vi "main.vi"(0 "Power":bool, 1 "Bean level":dbl(slide) scale=0.0..100.0, 2 "Milk level":dbl(slide) scale=0.0..100.0, 5 "1 Cup":bool, 7 "1 Carafe":bool, 8 "Chamber":dbl(slide) scale=0.0..60.0, 9 "Water level":dbl(slide) scale=0.0..100.0, 10 "Dispenser":dbl(slide) scale=0.0..60.0, 11 "Error in":errorcluster) -> (4 "Elapsed Time":dbl, 6 "Total Cups":dbl, 12 "Low Water":bool, 13 "Low Bean":bool, 14 "Low Milk":bool, 15 "Error out":errorcluster)   [LabVIEW 2020, in "coffee machine.lvlib"]
doc: "This system is a coffee maker which can be produce variety of coffees based on the user input."
uses:
  coffee machine.lvlib
  Typedefs/Queue operations.ctl
  Typedefs/Data cluster.ctl
  <vilib>/Utility/config.llb/Write Key (String).vi
  <vilib>/Utility/config.llb/NI_LVConfig.lvlib
panel:
  out "Previous time":dbl
  out "Dispensing":bool
  out "Brewing":bool
  out "Grinding":bool
  out "Heating":bool
  out "Purging":bool
  in  "Select drink":dbl(knob) scale=0.0..10.0
  # "Coffee"
  # "Latte"
  # "Hot water"
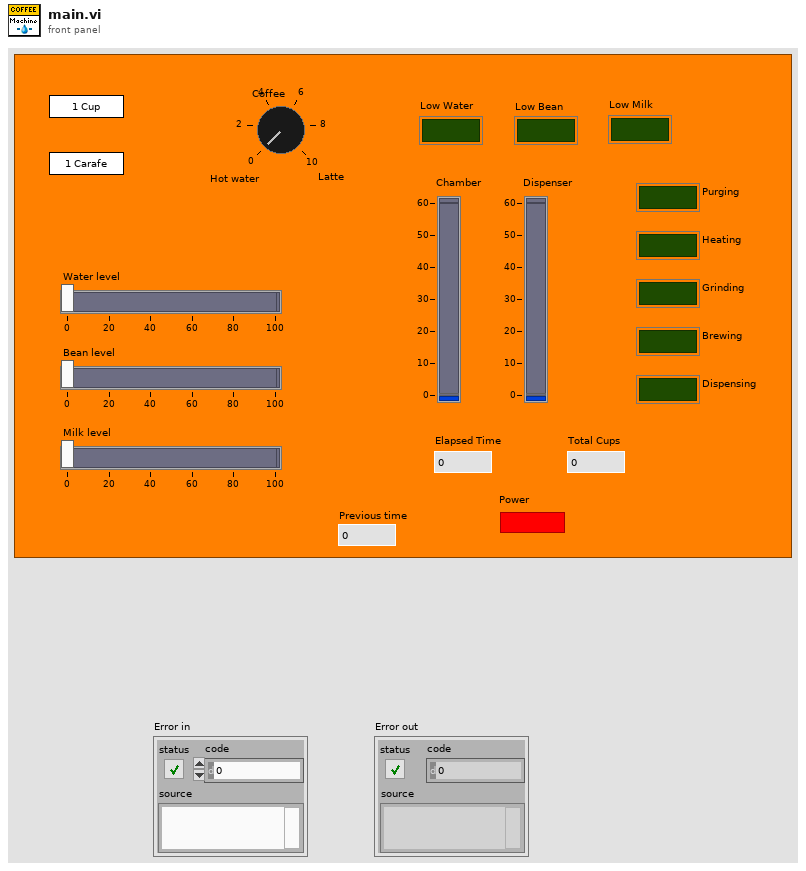
[diagram p1: front panel]
types:
  T1 = typedef "Data cluster.ctl" = cluster{"Timing":cluster{"Start time":dbl, "Elapsed time":dbl, "Previous time":dbl, "Started":bool, "Paused":bool}, "Enable controls":refnum<vi>[], "Disable controls":refnum<vi>[], "Low Water":bool, "Low Bean":bool, "Low Milk":bool, "Purging":bool, "Heating":bool, "Grinding":bool, "Brewing":bool, "Dispensing":bool, "Elapsed time":dbl, "Total Cups":dbl, "Path":path}
  T2 = typedef "coffee machine.lvlib/Queue operations.ctl" = enum16{"Create queue", " Enqueue N", "Enstack N", "Dequeue", "Flush", "Release", ""}
  T3 = cluster{"Start time":dbl, "Elapsed time":dbl, "Previous time":dbl, "Started":bool, "Paused":bool}
  T4 = typedef "NI_LVConfig.lvlib/Config Data RefNum.ctl" = refnum<k1>
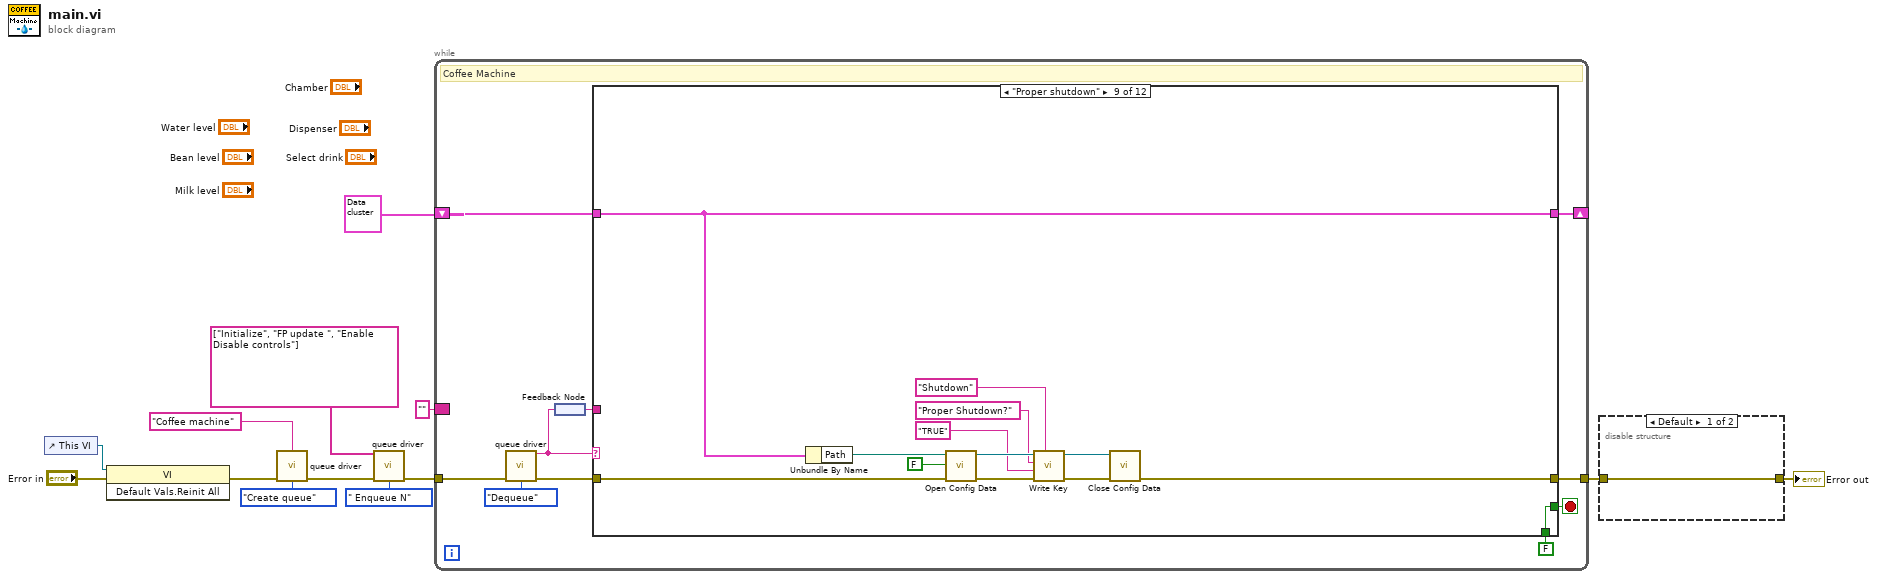
[diagram p0: block diagram]
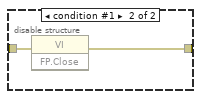
[diagram p2: hidden frame]
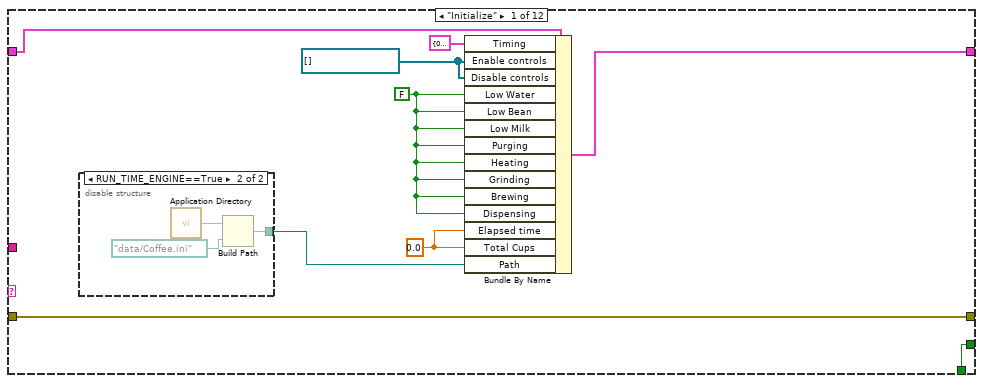
[diagram p3: hidden frame]
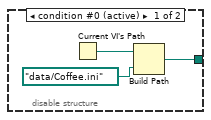
[diagram p4: hidden frame]
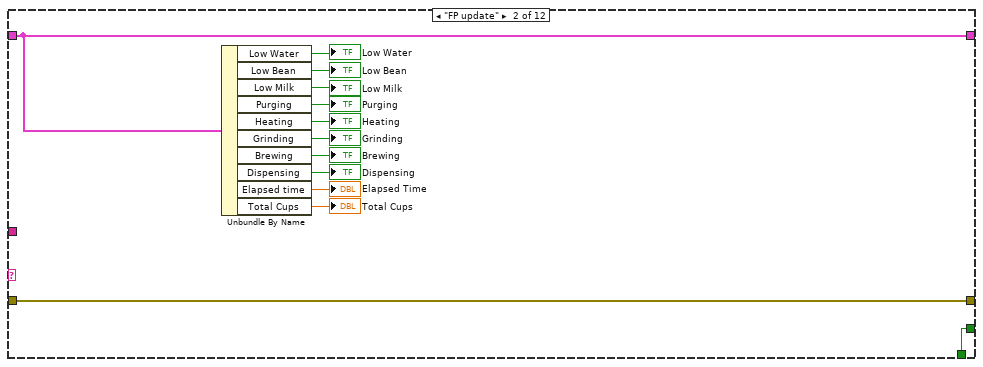
[diagram p5: hidden frame]
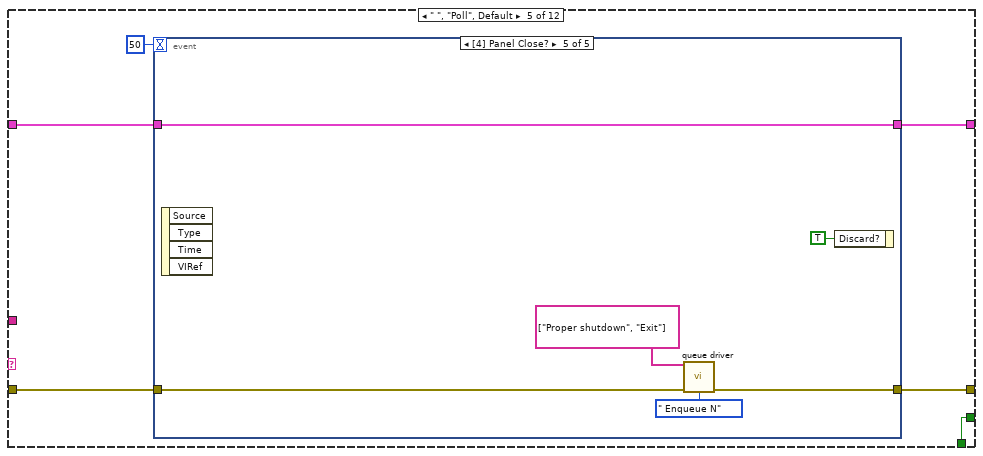
[diagram p8: hidden frame]
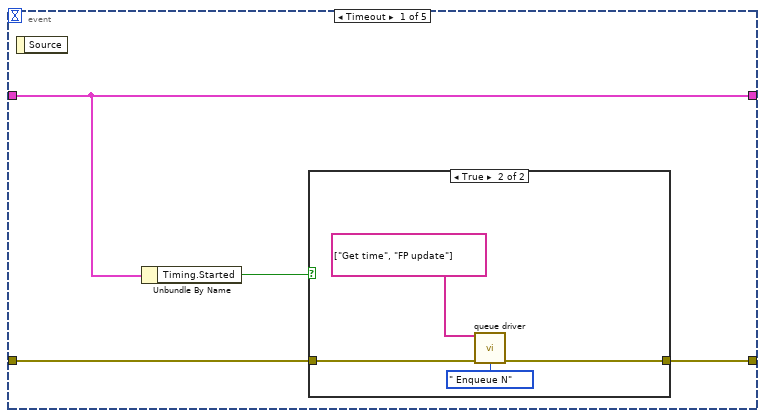
[diagram p9: hidden frame]
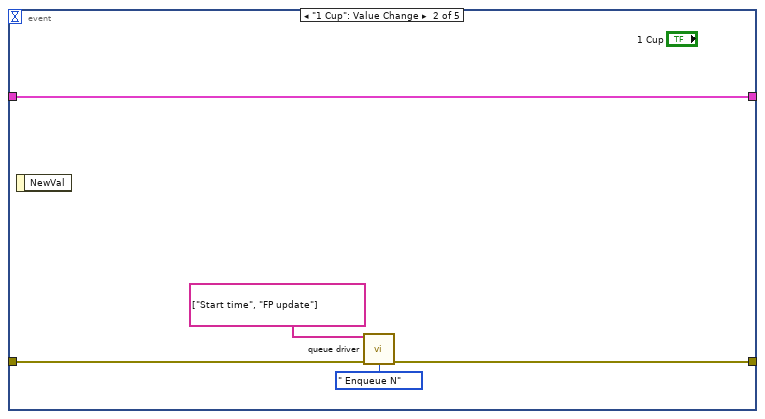
[diagram p11: hidden frame]
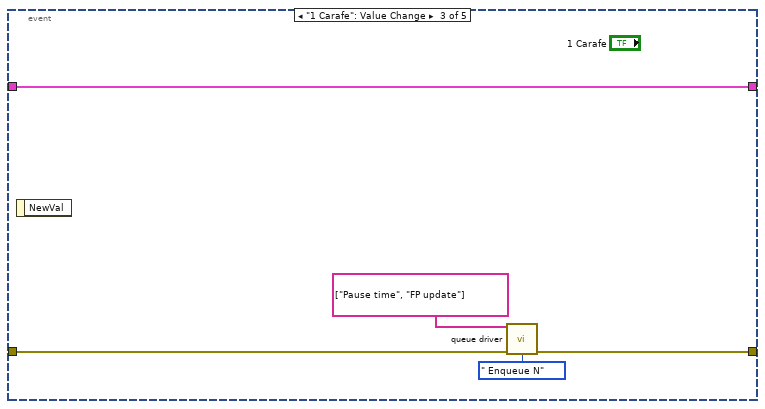
[diagram p12: hidden frame]
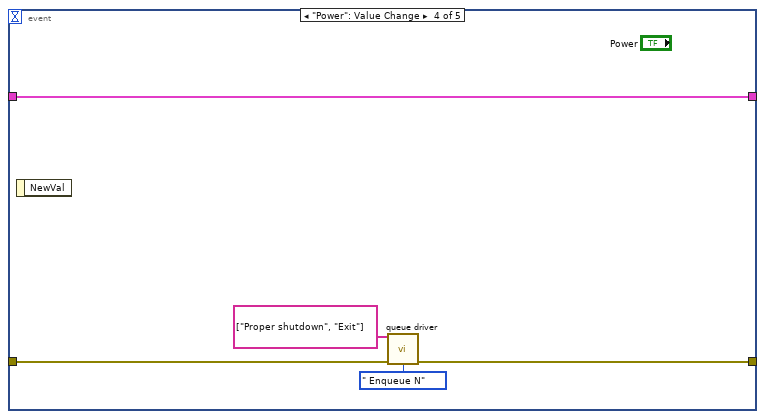
[diagram p13: hidden frame]
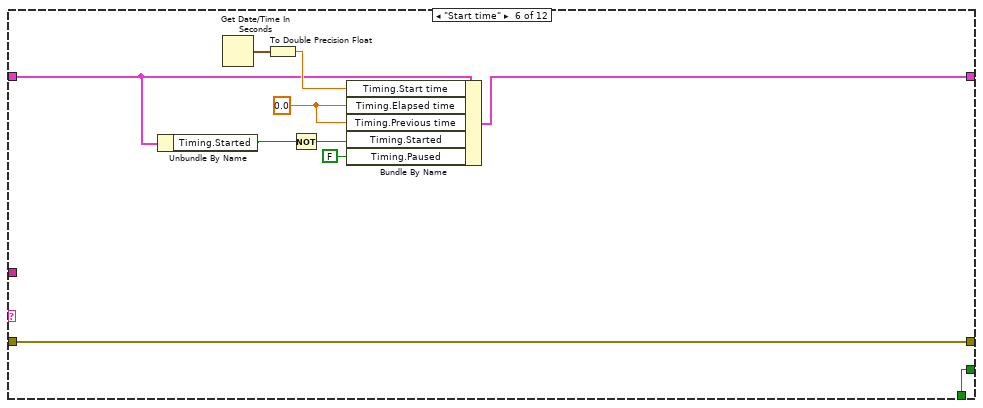
[diagram p14: hidden frame]
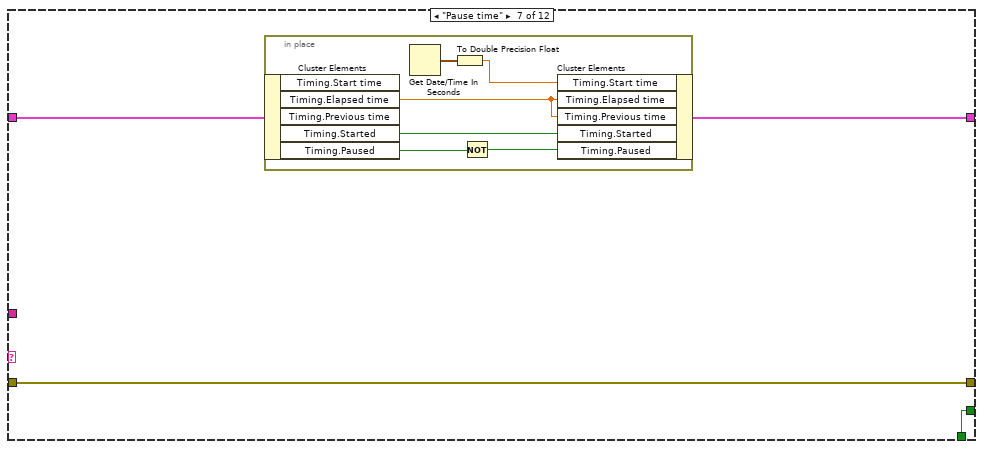
[diagram p15: hidden frame]
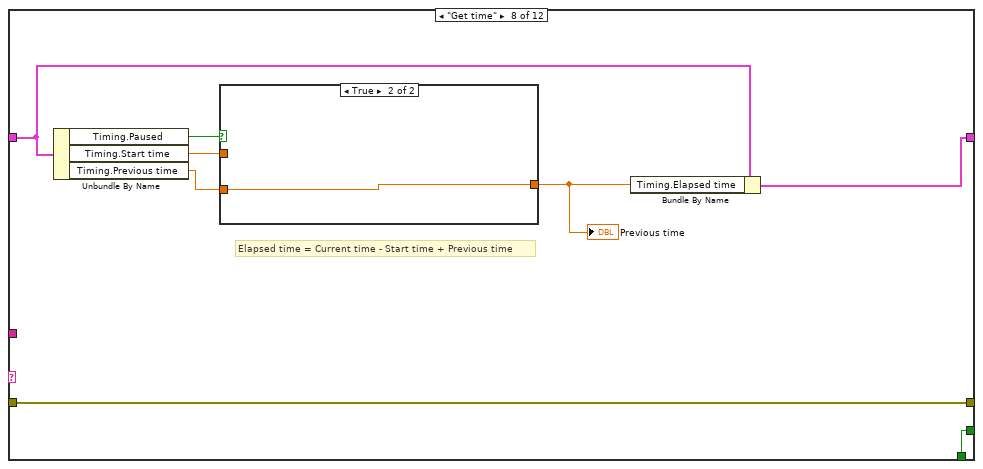
[diagram p16: hidden frame]
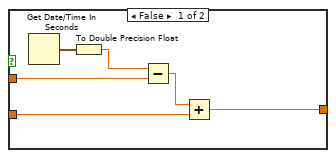
[diagram p17: hidden frame]
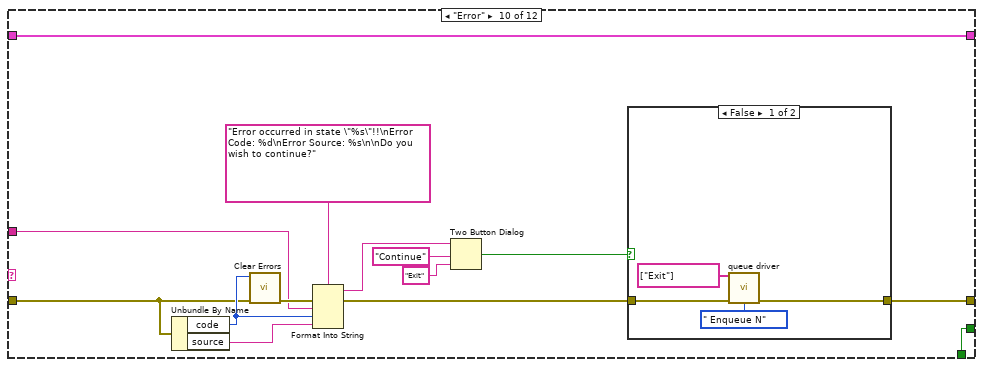
[diagram p18: hidden frame]
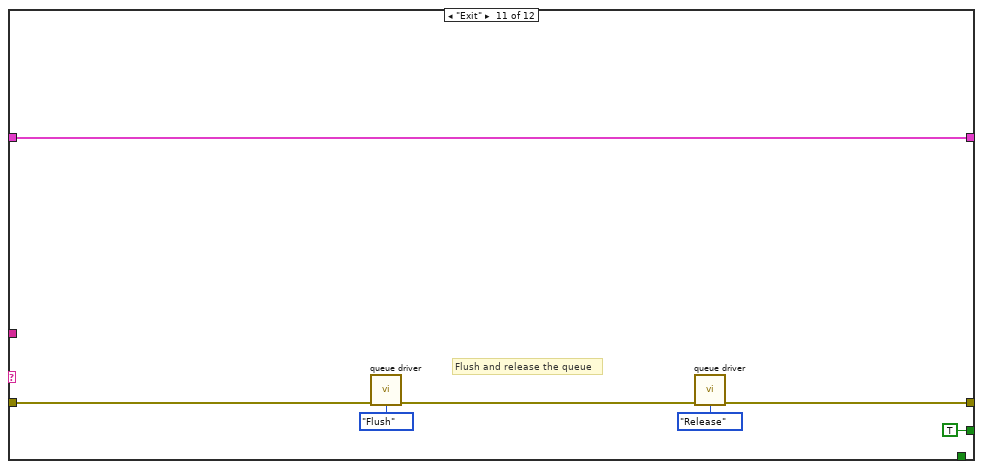
[diagram p20: hidden frame]
diagram:
  n1 = control-ref of="This VI"() -> (w11:refnum<vi>)
  n2 = invoke class="VI" method="Default Vals.Reinit All"(reference=w11, error in="Error in") -> (error out=w10:errorcluster)  [unwired: 1 in, 2 out]
  n3 = call "queue driver.vi"("Name"="Coffee machine", "Error in"=w10, "Queue operations"=Queue_operations."Create queue") -> ("Error out"=w7:errorcluster)  [unwired: 11 in, 1 out]
  n4 = call "queue driver.vi"("Enqueue"=string[] ["Initialize", "FP update ", "Enable Disable controls"], "Error in"=w7, "Queue operations"=Queue_operations." Enqueue N") -> ("Error out"=w5:errorcluster)  [unwired: 11 in, 1 out]
  n5 = while {
    tunnel: w5 -> [w20]
    border: "" ("Dequeued element") -> [_]
    shift-right: [w15] -> _
    shift-left: T1 {"Timing"={"Start time"=0.0, "Elapsed time"=0.0, "Previous time"=0.0, "Started"=FALSE, "Paused"=FALSE}, "Enable controls"=[], "Disable controls"=[], "Low Water"=FALSE, "Low Bean"=FALSE, "Low Milk"=FALSE, "Purging"=FALSE, "Heating"=FALSE, "Grinding"=FALSE, "Brewing"=FALSE, "Dispensing"=FALSE, "Elapsed time"=0.0, "Total Cups"=0.0, "Path"=path ""} -> [w14]
    tunnel: [w16] -> w2
    stop <- w23 stop-if-true
    # "Coffee Machine"
    n6 = call "queue driver.vi"("Error in"=w20, "Queue operations"=Queue_operations."Dequeue") -> ("Dequeued element"=w19:string, "Error out"=w17:errorcluster)  [unwired: 12 in]
    n7 = feedback-in #1(w19) -> ()
    n8 = feedback #1() -> (w18:string)
    n9 = case shown="\"Proper shutdown\"" w19 {
      tunnel: [w32 w51 w54 w57 w63 w103 w107 w121 w141 w155 TRUE w170] -> w23
      tunnel: FALSE -> [w32 w51 w54 w57 w63 w103 w107 w121 w141 w155 _ w170]
      tunnel: w18 -> [_ _ _ _ _ _ _ _ _ w146 _ _]
      tunnel: w17 -> [w31 w50 w53 w56 w62 w102 w106 w120 w140 w147 w165 w169]
      tunnel: [w31 w50 w53 w56 w61 w102 w106 w120 w130 w143 w163 w169] -> w16
      tunnel: [w25 w39 w52 w55 w59 w101 w104 w114 w129 w142 w161 w168] -> w15
      tunnel: w14 -> [w30 w39 w52 w55 w58 w96 w105 w116 w129 w142 w161 w168]
      frame "Initialize" {
        w26 = 0.0 ("Total Cups")
        w27 = FALSE ("Low Water")
        w28 = refnum<vi>[] [] ("Enable controls")
        n10 = disable-structure shown="RUN_TIME_ENGINE==True" {
          disable-tunnel: [w33 w37] -> w24
          frame condition #0 (active) {
            n11 = Current VI's Path() -> (path=w35:path)
            n12 = Build Path(base path=w35, name or relative path=path "data/Coffee.ini") -> (appended path=w33:path)
          }
          frame condition #1 {
            n13 = call <vilib>:"Application Directory.vi"() -> ("Application Directory"=w36:path)
            n14 = Build Path(base path=w36, name or relative path=path "data/Coffee.ini") -> (appended path=w37:path)
          }
        }
        n15 = Bundle By Name(cluster=w30, "Timing"=T3 {"Start time"=0.0, "Elapsed time"=0.0, "Previous time"=0.0, "Started"=FALSE, "Paused"=FALSE}, "Enable controls"=w28, "Disable controls"=w28, "Low Water"=w27, "Low Bean"=w27, "Low Milk"=w27, "Purging"=w27, "Heating"=w27, "Grinding"=w27, "Brewing"=w27, "Dispensing"=w27, "Elapsed time"=w26, "Total Cups"=w26, "Path"=w24) -> (w25:T1)
      }
      frame "FP update" {
        n16 = Unbundle By Name(w39) -> ("Low Water"=→"Low Water":bool, "Low Bean"=→"Low Bean":bool, "Low Milk"=→"Low Milk":bool, "Purging"=→"Purging":bool, "Heating"=→"Heating":bool, "Grinding"=→"Grinding":bool, "Brewing"=→"Brewing":bool, "Dispensing"=→"Dispensing":bool, "Elapsed time"=→"Elapsed Time":dbl, "Total Cups"=→"Total Cups":dbl)
      }
      frame "Enable Disable controls" {
      }
      frame "Read and write file" {
      }
      frame " ", "Poll", Default {
        n17 = event shown="[4] Panel Close?" {
          selector: _ -> [_ _ _ _ _]
          dyn-events: _ -> [_ _ _ _ _]
          timeout: 50 -> [_ _ _ _ _]
          tunnel: w62 -> [w65 w75 w79 w85 w89]
          tunnel: [w64 w74 w78 w84 w88] -> w61
          tunnel: [w67 w77 w82 w87 w93] -> w59
          tunnel: w58 -> [w67 w77 w82 w87 w93]
          event Timeout {
            n18 = event-data() -> ()  [unwired: 1 in, 1 out]
            n19 = Unbundle By Name(w67) -> ("Timing.Started"=w66:bool)
            n20 = case shown="True" w66 {
              tunnel: w65 -> [w68 w71]
              tunnel: [w68 w70] -> w64
              frame False {
              }
              frame True {
                n21 = call "queue driver.vi"("Enqueue"=string[] ["Get time", "FP update"], "Error in"=w71, "Queue operations"=Queue_operations." Enqueue N") -> ("Error out"=w70:errorcluster)  [unwired: 11 in, 1 out]
              }
            }
          }
          event "1 Cup": Value Change {
            n22 = event-data() -> ()  [unwired: 1 in, 1 out]
            n23 = call "queue driver.vi"("Enqueue"=string[] ["Start time", "FP update"], "Error in"=w75, "Queue operations"=Queue_operations." Enqueue N") -> ("Error out"=w74:errorcluster)  [unwired: 11 in, 1 out]
          }
          event "1 Carafe": Value Change {
            n24 = event-data() -> ()  [unwired: 1 in, 1 out]
            n25 = call "queue driver.vi"("Enqueue"=string[] ["Pause time", "FP update"], "Error in"=w79, "Queue operations"=Queue_operations." Enqueue N") -> ("Error out"=w78:errorcluster)  [unwired: 11 in, 1 out]
          }
          event "Power": Value Change {
            n26 = event-data() -> ()  [unwired: 1 in, 1 out]
            n27 = call "queue driver.vi"("Enqueue"=string[] ["Proper shutdown", "Exit"], "Error in"=w85, "Queue operations"=Queue_operations." Enqueue N") -> ("Error out"=w84:errorcluster)  [unwired: 11 in, 1 out]
          }
          event Panel Close? {
            n28 = event-data() -> ()  [unwired: 1 in, 4 out]
            n29 = call "queue driver.vi"("Enqueue"=string[] ["Proper shutdown", "Exit"], "Error in"=w89, "Queue operations"=Queue_operations." Enqueue N") -> ("Error out"=w88:errorcluster)  [unwired: 11 in, 1 out]
            n30 = event-data("Discard?"=TRUE) -> ()  [unwired: 1 in, 1 out]
          }
        }
      }
      frame "Start time" {
        w98 = 0.0 ("Timing.Elapsed time")
        n31 = Unbundle By Name(w96) -> ("Timing.Started"=w94:bool)
        n32 = Get Date/Time In Seconds() -> (seconds since 1Jan1904=w100:timestamp)
        n33 = To Double Precision Float(number=w100) -> (double precision float=w99:dbl)
        n34 = Not(x=w94) -> (.not. x?=w95:bool)
        n35 = Bundle By Name(cluster=w96, "Timing.Start time"=w99, "Timing.Elapsed time"=w98, "Timing.Previous time"=w98, "Timing.Started"=w95, "Timing.Paused"=FALSE) -> (w101:T1)
      }
      frame "Pause time" {
        n36 = in-place {
          n37 = in-place-cluster #2(w105) -> ("Timing.Elapsed time"=w109:dbl, "Timing.Started"=w108:bool, "Timing.Paused"=w111:bool)  [unwired: 2 out]
          n38 = Get Date/Time In Seconds() -> (seconds since 1Jan1904=w113:timestamp)
          n39 = To Double Precision Float(number=w113) -> (double precision float=w112:dbl)
          n40 = Not(x=w111) -> (.not. x?=w110:bool)
          n41 = in-place-cluster #2("Timing.Start time"=w112, "Timing.Elapsed time"=w109, "Timing.Previous time"=w109, "Timing.Started"=w108, "Timing.Paused"=w110) -> (w104:T1)
        }
      }
      frame "Get time" {
        # "Elapsed time = Current time - Start time + Previous time"
        n42 = Unbundle By Name(w116) -> ("Timing.Paused"=w119:bool, "Timing.Start time"=w118:dbl, "Timing.Previous time"=w117:dbl)
        n43 = case shown="True" w119 {
          tunnel: w118 -> [w125 _]
          tunnel: w117 -> [w123 w128]
          tunnel: [w122 w128] -> w115
          frame False {
            n44 = Get Date/Time In Seconds() -> (seconds since 1Jan1904=w127:timestamp)
            n45 = To Double Precision Float(number=w127) -> (double precision float=w126:dbl)
            n46 = Subtract(x=w126, y=w125) -> (x-y=w124:dbl)
            n47 = Add(x=w124, y=w123) -> (x+y=w122:dbl)
          }
          frame True {
          }
        }
        "Previous time" <- w115
        n48 = Bundle By Name(cluster=w116, "Timing.Elapsed time"=w115) -> (w114:T1)
      }
      frame "Proper shutdown" {
        n49 = Unbundle By Name(w129) -> ("Path"=w137:path)
        n50 = call <vilib>:"Open Config Data.vi"("error in (no error)"=w140, "create file if necessary (T)"=FALSE, "configuration file path"=w137) -> ("error out"=w139:errorcluster, "refnum"=w135:T4)  [unwired: 6 in, 1 out]
        n51 = call-poly <vilib>:"Write Key.vi"("section"="Shutdown", "error in (no error)"=w139, "value"="TRUE", "key"="Proper Shutdown?", "refnum"=w135) -> ("error out"=w138:errorcluster, "refnum out"=w132:T4)  [unwired: 4 in, 1 out]
        n52 = call <vilib>:"Close Config Data.vi"("error in (no error)"=w138, "refnum"=w132) -> ("error out"=w130:errorcluster)  [unwired: 8 in, 1 out]
      }
      frame "Error" {
        n53 = Unbundle By Name(w147) -> ("code"=w152:i32, "source"=w151:string)
        n54 = call <vilib>:"Clear Errors.vi"("error in (no error)"=w147, "specific error code to clear (0: all)"=w152) -> ("error out"=w154:errorcluster)  [unwired: 4 in, 1 out]
        n55 = Format Into String(format string="Error occurred in state \"%s\"!!\nError Code: %d\nError Source: %s\n\nDo you wish to continue?", error in=w154, w146, w152, w151) -> (resulting string=w150:string, error out=w145:errorcluster)  [unwired: 1 in]
        n56 = Two Button Dialog(message=w150, 1:"Exit" ("F button name (\"Cancel\")"), 2:"Continue" ("T button name (\"OK\")")) -> (T button?=w144:bool)
        n57 = case shown="False" w144 {
          tunnel: w145 -> [w158 w160]
          tunnel: [w157 w160] -> w143
          frame False {
            n58 = call "queue driver.vi"("Enqueue"=string[] ["Exit"], "Error in"=w158, "Queue operations"=Queue_operations." Enqueue N") -> ("Error out"=w157:errorcluster)  [unwired: 11 in, 1 out]
          }
          frame True {
          }
        }
      }
      frame "Exit" {
        # "Flush and release the queue"
        n59 = call "queue driver.vi"("Error in"=w165, "Queue operations"=Queue_operations."Flush") -> ("Error out"=w164:errorcluster)  [unwired: 12 in, 1 out]
        n60 = call "queue driver.vi"("Error in"=w164, "Queue operations"=Queue_operations."Release") -> ("Error out"=w163:errorcluster)  [unwired: 12 in, 1 out]
      }
      frame "Developer error" {
      }
    }
  }
  n61 = disable-structure shown="Default" {
    disable-tunnel: w2 -> [w171 w173]
    disable-tunnel: [w171 w172] -> w1
    frame condition #0 (active) {
    }
    frame condition #1 {
      n62 = invoke class="VI" method="FP.Close"(error in=w173) -> (error out=w172:errorcluster)  [unwired: 2 in, 2 out]
    }
  }
  "Error out" <- w1
